vi "switch.vi"(9 "switch":bool=TRUE, 10 "toggle":bool=TRUE) -> (1 "result":bool=TRUE, 2 "toggle out":bool=TRUE)   [LabVIEW 2010]
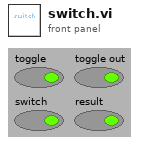
[diagram p1: front panel]
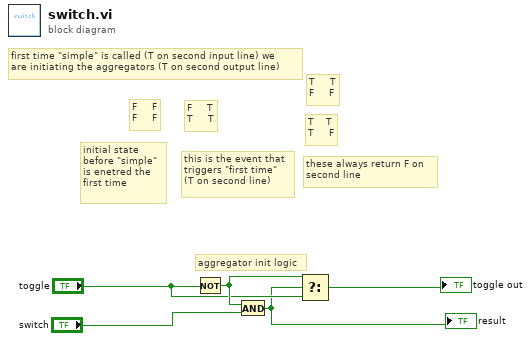
[diagram p0: block diagram]
diagram:
  # "these always return F on \nsecond line"
  # "initial state\nbefore \"simple\"\nis enetred the \nfirst time"
  # "this is the event that \ntriggers \"first time\" \n(T on second line)"
  # "F     F\nF     F"
  # "T     T\nF     F"
  # "F     T\nT     T"
  # "T    T\nT     F"
  # "first time \"simple\" is called (T on second input line) we \nare initiating the aggregators (T on second output line)"
  # "aggregator init logic"
  n1 = Not(x="toggle") -> (.not. x?=w5:bool)
  n2 = And(x=w5, y="switch") -> (x .and. y?=w1:bool)
  "result" <- w1
  n3 = Select(t=w5, s=w1, f="toggle") -> (s? t:f=→"toggle out":bool)
